vi "validate line configuration.vi"(7 "module":refnum<class "Tagbus PID Module configuration.lvclass">, 11 "line in":T1={"ID"="", "Setpoint"=refnum, "Process Variable"=refnum, "Output"=refnum, "PID gains"={"proportional gain (Kc)"=1.0, "integral time (Ti, min)"=0.01, "derivative time (Td, min)"=0.0}, "output range"={"output high"=100.0, "output low"=-100.0}} {"output range"."output low" format="%.2f"; "output range"."output high" format="%.2f"; "PID gains"."proportional gain (Kc)" format="%.2f"; "PID gains"."integral time (Ti, min)" format="%.2f"}) -> (1 "valid?":bool, 2 "errors":string, 3 "line out":T1={"ID"="", "Setpoint"=refnum, "Process Variable"=refnum, "Output"=refnum, "PID gains"={"proportional gain (Kc)"=1.0, "integral time (Ti, min)"=0.01, "derivative time (Td, min)"=0.0}, "output range"={"output high"=100.0, "output low"=-100.0}} {"output range"."output low" format="%.2f"; "output range"."output high" format="%.2f"; "PID gains"."proportional gain (Kc)" format="%.2f"; "PID gains"."integral time (Ti, min)" format="%.2f"})   [LabVIEW 2014, in "Tagbus PID Module editor node.lvclass"]
uses:
  Tagbus PID Module editor node.lvclass
  table line.ctl
  <vilib>/NI/Tag Bus Module Framework/channel/TBM channel.lvclass
  module/configuration/Tagbus PID Module configuration.lvclass
  <vilib>/NI/Tag Bus/tag/tag descriptor.lvclass/tag descriptor.ctl
  <vilib>/NI/Tag Bus/tag/read tag name.vi
  <vilib>/NI/Tag Bus/tag/read data type.vi
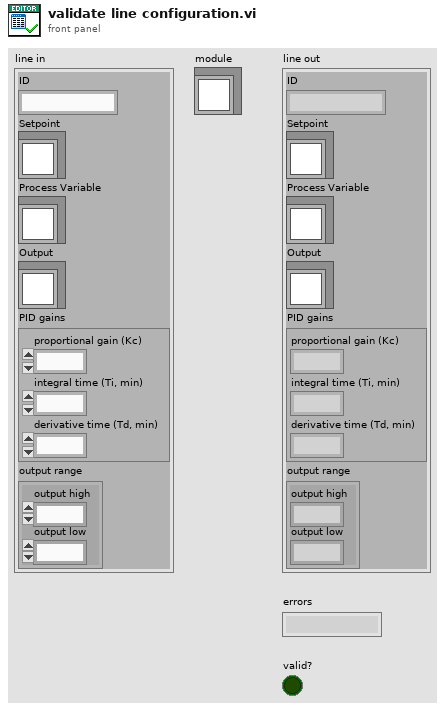
[diagram p1: front panel]
types:
  T1 = typedef "Tagbus PID Module editor node.lvclass/table line.ctl" = cluster{"ID":string, "Setpoint":refnum<class "TBM channel.lvclass">, "Process Variable":refnum<class "TBM channel.lvclass">, "Output":refnum<class "TBM channel.lvclass">, "PID gains":cluster{"proportional gain (Kc)":dbl, "integral time (Ti, min)":dbl, "derivative time (Td, min)":dbl}, "output range":cluster{"output high":dbl, "output low":dbl}}
  T2 = typedef "tag bus.lvlib/tag descriptor.lvclass/Data Type.ctl" = enum16{"Double", "Single", "I64", "I32", "I16", "I8", "U64", "U32", "U16", "U8", "Boolean", "String", "Array of Double", "Array of Single", "Array of I64", "Array of I32", "Array of I16", "Array of I8", "Array of U64", "Array of U32", "Array of U16", "Array of U8", "Array of Boolean", "Array of String"}
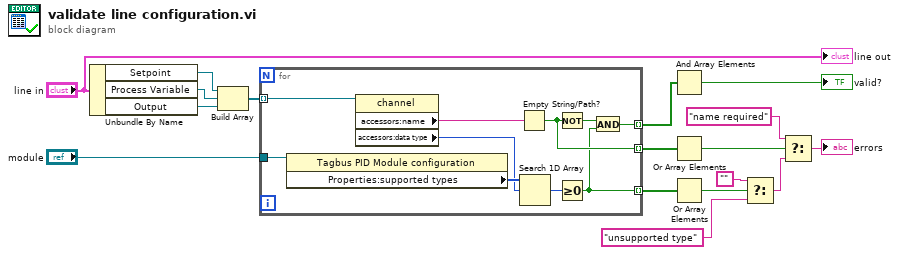
[diagram p0: block diagram]
diagram:
  n1 = Unbundle By Name("line in") -> ("Setpoint"=w10:refnum<class "TBM channel.lvclass">, "Process Variable"=w9:refnum<class "TBM channel.lvclass">, "Output"=w8:refnum<class "TBM channel.lvclass">)
  n2 = Build Array(w10, w9, w8) -> (w7:refnum<class "TBM channel.lvclass">[])
  n3 = for {
    tunnel: "module" -> [w25]
    tunnel: [w22] -> w6 mode=indexing
    tunnel: [w20] -> w4 mode=indexing
    tunnel: [w19] -> w2 mode=indexing
    tunnel: w7 -> [w18] mode=indexing
    n4 = property class="Tagbus PID Module configuration"(reference=w25) -> ("Properties:supported types"=w24:T2[])  [unwired: 1 in, 2 out]
    n5 = property class="channel"(reference=w18) -> ("accessors:name"=w27:string, "accessors:data type"=w23:T2)  [unwired: 1 in, 2 out]
    n6 = Empty String/Path?(string/path=w27) -> (empty?=w20:bool)
    n7 = Search 1D Array(1D array=w24, element=w23) -> (index of element=w21:i32)  [unwired: 1 in]
    n8 = Not(x=w20) -> (.not. x?=w26:bool)
    n9 = Greater Or Equal To 0?(x=w21) -> (x >= 0?=w19:bool)
    n10 = And(x=w26, y=w19) -> (x .and. y?=w22:bool)
  }
  n11 = And Array Elements(Boolean array=w6) -> (logical AND=→"valid?":bool)
  n12 = Or Array Elements(Boolean array=w4) -> (logical OR=w3:bool)
  n13 = Or Array Elements(Boolean array=w2) -> (logical OR=w1:bool)
  n14 = Select(t="", s=w1, f="unsupported type") -> (s? t:f=w12:string)
  n15 = Select(t="name required", s=w3, f=w12) -> (s? t:f=→"errors":string)
  "line out" <- "line in"
